vi "capture.vi"(6 "error in (no error)":errorcluster, 7 "Cam ID":u32, 8 "Image in":T1, 9 "session in":refnum<k35>) -> (0 "error out":errorcluster, 2 "Image out":T1, 3 "session out":refnum<k35>)   [LabVIEW 2022 SP3]
uses:
  <vilib>/vision/Image Controls.llb/IMAQ Image.ctl
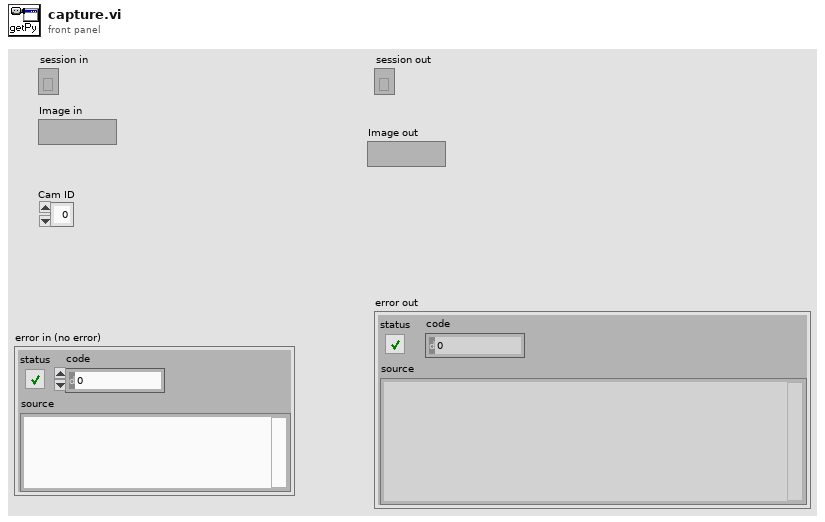
[diagram p1: front panel]
types:
  T1 = typedef "IMAQ Image.ctl" = refnum<image>
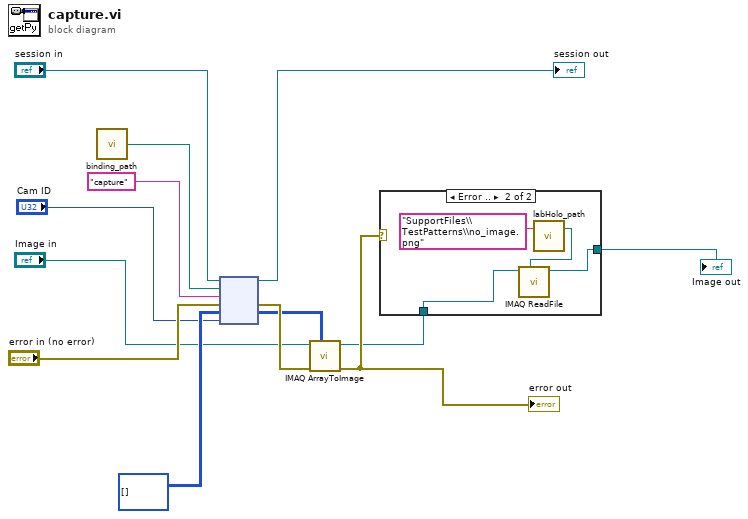
[diagram p0: block diagram]
diagram:
  n1 = call "binding_path.vi"() -> ("appended path"=w7:path)
  n2 = node("session in", w7, "capture" ("function name"), "error in (no error)", u16[][] [] ("image"), "Cam ID") -> (→"session out":refnum<k35>, w9:errorcluster, w5:u16[][])  [unwired: 1 in, 2 out]
  n3 = call "IMAQ ArrayToImage"("Image Pixels (U16)"=w5, "error in (no error)"=w9, "Image"="Image in") -> ("error out"=w3:errorcluster, "Image Out"=w1:T1)  [unwired: 7 in]
  "error out" <- w3
  n4 = case shown="Error .." w3 {
    tunnel: [w14 w16] -> w2
    tunnel: w1 -> [w14 w17]
    frame No Error {
    }
    frame Error {
      n5 = call "labHolo_path.vi"("sub folder or file (str)"="SupportFiles\\TestPatterns\\no_image.png") -> ("labHolo path"=w15:path)  [unwired: 1 in, 1 out]
      n6 = call "IMAQ ReadFile"("File Path"=w15, "Image"=w17) -> ("Image Out"=w16:T1)  [unwired: 5 in, 4 out]
    }
  }
  "Image out" <- w2
